vi "Init Condition.vi"(5 "Sequencing":refnum<class "MessageQ.lvclass">, 6 "Variables":refnum<class "Variables.lvclass">, 7 "VolatusAPI":refnum<class "VolatusAPI.lvclass">, 8 "error in (no error)":refnum<class "MultiErrors.lvclass">, 10 "Condition Config":refnum<class "Condition Config.lvclass">, 11 "LowLimit Condition in":refnum<class "LowLimit Condition.lvclass">) -> (0 "error out":refnum<class "MultiErrors.lvclass">, 3 "LowLimit Condition out":refnum<class "LowLimit Condition.lvclass">)   [LabVIEW 2020, in "VolatusSeq.lvlib" / "LowLimit Condition.lvclass"]
uses:
  LowLimit Condition.lvclass
  VolatusErrorUtilities/MultiErrors/MultiErrors.lvclass
  Volatus/VolatusAPI/VolatusAPI.lvclass
  VolatusSeqConfig/Condition Config/Condition Config.lvclass
  Volatus/MessageQ/MessageQ.lvclass
  VolatusSeqConfig/LowLimit Condition Config/LowLimit Condition Config.lvclass
  VolatusSeqConfig/LowLimit Condition Config/LowLimit Condition Config.lvclass/LowLimit Condition Config.ctl
  Volatus/VolatusAPI/VolatusAPI.lvclass/VolatusAPI.ctl
  LowLimit Condition.lvclass/LowLimit Condition.ctl
  lv-vecto/Vecto/ChannelService/Lookup Double Channel.vi
  Condition Value/Condition Value.lvclass
  Variables/Variables.lvclass
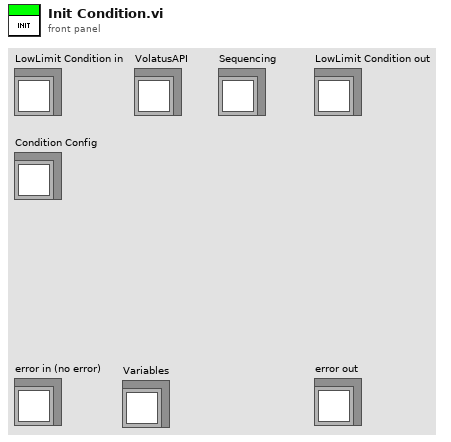
[diagram p1: front panel]
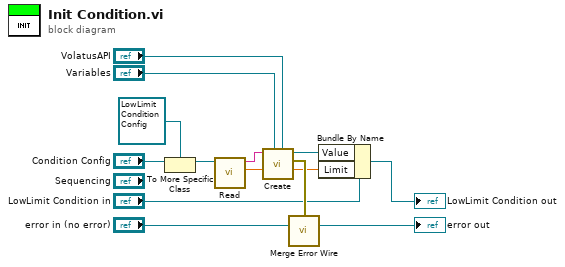
[diagram p0: block diagram]
diagram:
  n1 = To More Specific Class(target class=refnum<class "LowLimit Condition Config.lvclass"> refnum ("VolatusSeqConfig.lvlib:LowLimit Condition Config.lvclass"), reference="Condition Config") -> (specific class reference=w8:refnum<class "LowLimit Condition Config.lvclass">)  [unwired: 1 in, 1 out]
  n2 = call "Read.vi"("LowLimit Condition Config in"=w8) -> ("Limit"=w6:dbl, "Channel"=w4:string)  [unwired: 9 in]
  n3 = call "Create.vi"("VolatusAPI"="VolatusAPI", "Variables"="Variables", "Source Name"=w4) -> ("error out"=w13:errorcluster, "Condition Value out"=w1:refnum<class "Condition Value.lvclass">)  [unwired: 7 in]
  n4 = call "Merge Error Wire.vi"("error in (no error)"=w13, "MultiErrors in"="error in (no error)") -> ("MultiErrors out"=→"error out":refnum<class "MultiErrors.lvclass">)  [unwired: 13 in]
  n5 = Bundle By Name(cluster="LowLimit Condition in", "Value"=w1, "Limit"=w6) -> (→"LowLimit Condition out":refnum<class "LowLimit Condition.lvclass">)
